vi "CPT Read_Write_FIFO 12.1.vi"(0 "Device No.":u16=336 format="%.0x", 5 "FifoNo":i16=1, 7 "Number of Elements":i32, 9 "Path Logging":path, 11 "Record":bool) -> (4 "Device No. out":u16 format="%.0x", 8 "Output Array":dbl[][](array[numeric]))   [LabVIEW 2015]
uses:
  <vilib>/Analysis/2dsp.llb/Decimate (continuous, DBL).vi
  <vilib>/Analysis/NI_AALPro.lvlib
panel:
  in  "Decimaing?":bool
  out "error out":errorcluster
  out "Path Logging":path
  in  "Decimation Factor":i32
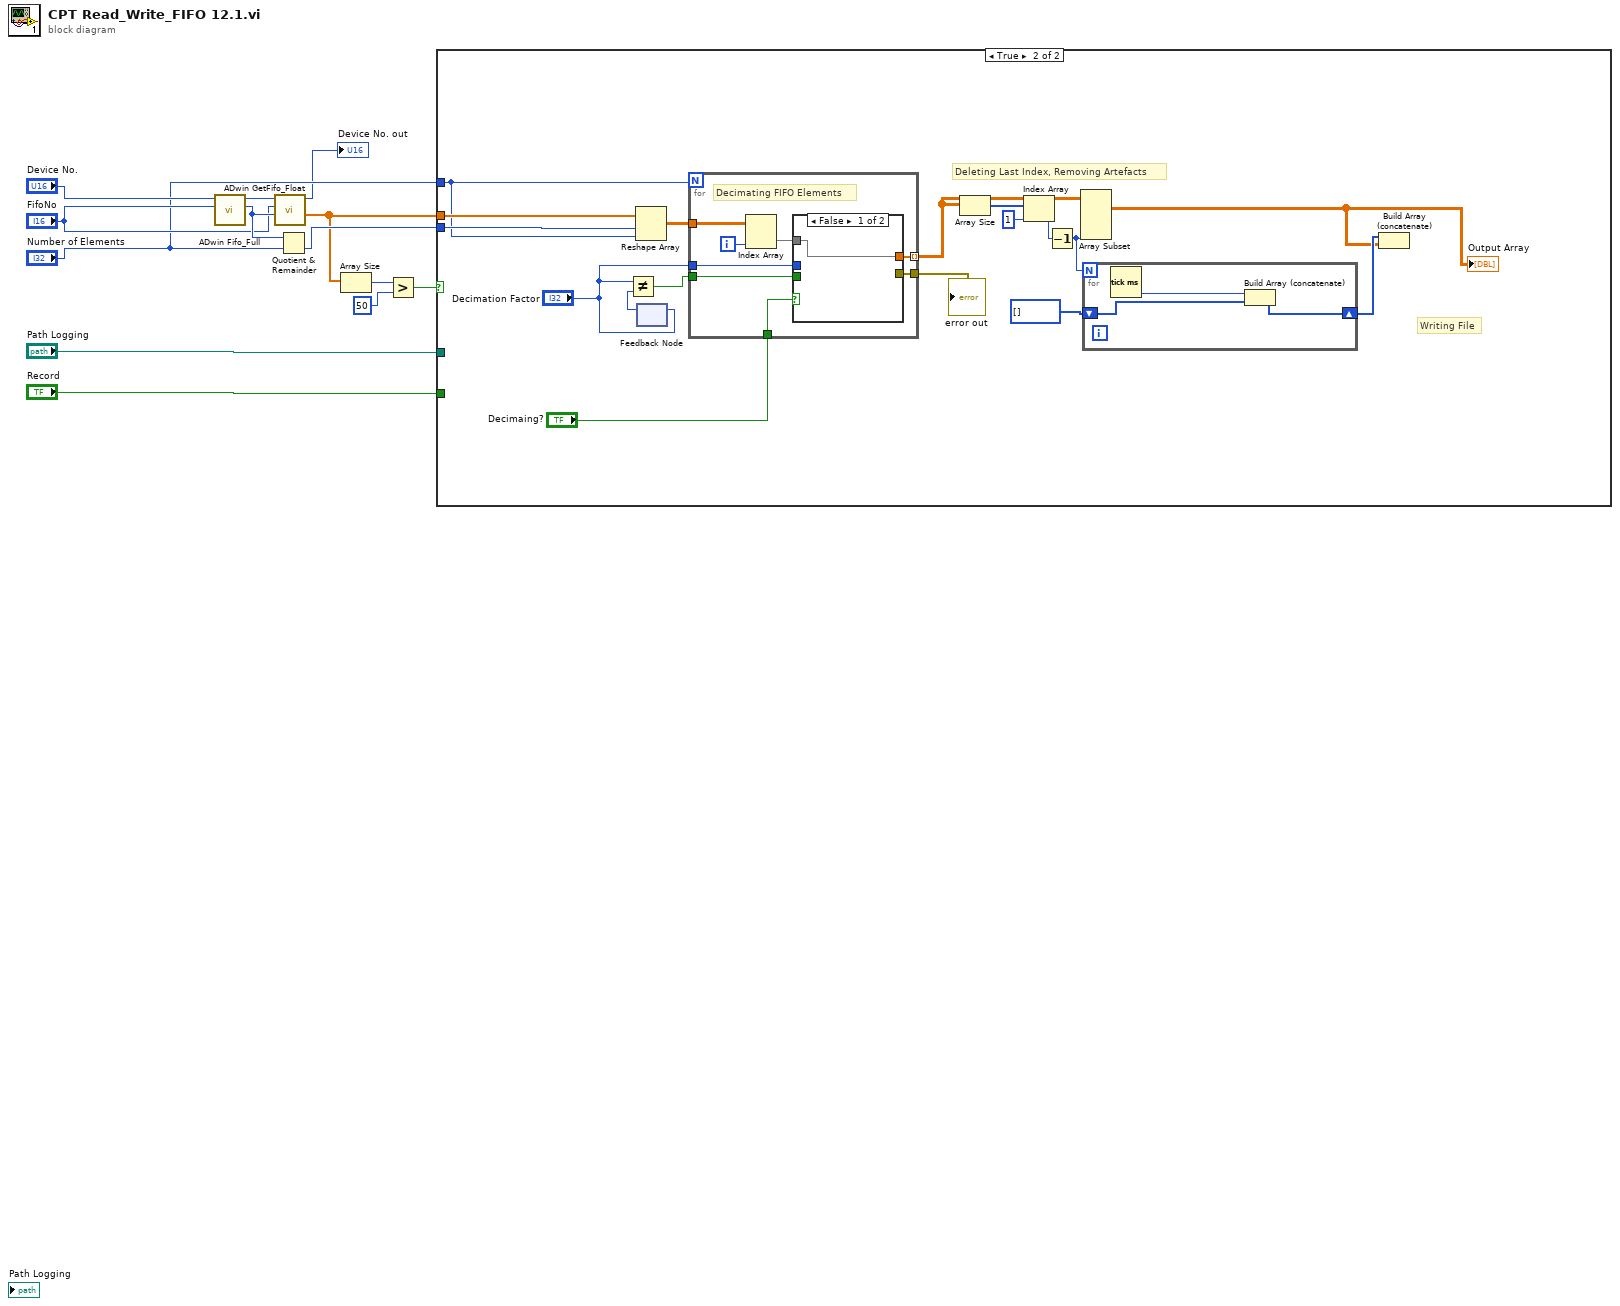
[diagram p0: block diagram]
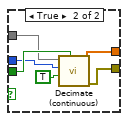
[diagram p3: hidden frame]
diagram:
  n1 = call "ADwin Fifo_Full.vi"("FifoNo"="FifoNo", "Device No."="Device No.") -> ("Count"=w12:i32, "Device No. out"=w11:u16)  [unwired: 7 in, 1 out]
  n2 = call "ADwin GetFifo_Float.vi"("count"=w12, "FifoNo"="FifoNo", "Device No."=w11) -> ("Data"=w4:sgl[], "Device No. out"=→"Device No. out":u16)  [unwired: 5 in, 2 out]
  n3 = Quotient & Remainder(x=w12, y="Number of Elements") -> (floor(x/y)=w13:i32)  [unwired: 1 out]
  n4 = Array Size(array=w4) -> (size(s)=w3:i32)
  n5 = Greater?(x=w3, y=50) -> (0:w2:bool)
  n6 = case shown="True" w2 {
    tunnel: w13 -> [_ w29]
    tunnel: w4 -> [_ w27]
    tunnel: "Record" -> [_ _]
    tunnel: "Path Logging" -> [_ _]
    tunnel: "Number of Elements" -> [_ w20]
    frame False {
    }
    frame True {
      # "Writing File"
      # "Deleting Last Index, Removing Artefacts"
      n7 = Reshape Array(w27, w29, w20) -> (w30:sgl[][])
      n8 = feedback #1() -> (w26:i32)  [unwired: 1 in]
      n9 = Not Equal?(x="Decimation Factor", y=w26) -> (x != y?=w25:bool)
      n10 = feedback-in #1("Decimation Factor") -> ()
      n11 = for {
        N: w20 -> [_]
        tunnel: w30 -> [w39]
        tunnel: w25 -> [w41]
        tunnel: "Decimation Factor" -> [w40]
        tunnel: [w37] -> w21 mode=indexing
        tunnel: [w35] -> w19
        tunnel: "Decimaing?" -> [w34]
        i -> [w38]
        # "Decimating FIFO Elements"
        n12 = Index Array(array=w39, index (col)=w38) -> (element=w36:sgl[])  [unwired: 1 in]
        n13 = case shown="False" w34 {
          tunnel: w41 -> [_ w48]
          tunnel: w40 -> [_ w46]
          tunnel: [w42 w45] -> w37
          tunnel: w36 -> [w42 w44]
          tunnel: [_ w43] -> w35
          frame False {
          }
          frame True {
            n14 = call-poly <vilib>:"Decimate (continuous).vi"("reset"=w48, "averaging"=TRUE, "decimating factor"=w46, "X"=w44) -> ("error out"=w43:errorcluster, "Decimated Array"=w45:dbl[])  [unwired: 6 in]
          }
        }
      }
      "error out" <- w19
      n15 = Array Size(array=w21) -> (size(s)=w24:i32[])
      n16 = Index Array(array=w24, index=1) -> (element=w22:i32)
      n17 = Decrement(x=w22) -> (x-1=w17:i32)
      n18 = Array Subset(array=w21, length (col)=w17) -> (w14:dbl[][])  [unwired: 3 in]
      "Output Array" <- w14
      n19 = for {
        N: w17 -> [_]
        shift-right: [w33] -> w15
        shift-left: u32[] [] -> [w31]
        n20 = Tick Count (ms)() -> (millisecond timer value=w32:u32)
        n21 = Build Array (concatenate)(w32, w31) -> (w33:u32[])
      }
      n22 = Build Array (concatenate)(w15, w14) -> ()  [unwired: 1 out]
    }
  }
